vi "Error Handler.vi"(8 "Error In":errorcluster) -> (0 "Error Out":errorcluster)   [LabVIEW 2019, in "Multisocket Example(Station1).lvlib"]
uses:
  Multisocket Example(Station1).lvlib
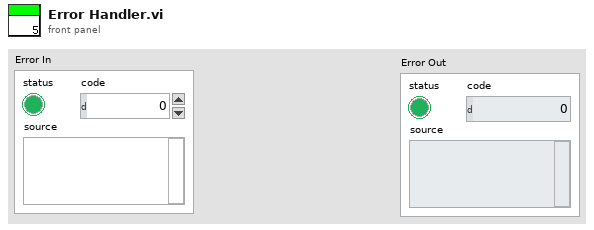
[diagram p1: front panel]
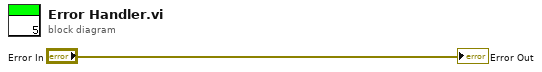
[diagram p0: block diagram]
diagram:
  "Error Out" <- "Error In"
